vi "Read Settings.vi"() -> (2 "Poly VI Paths":path[](array[path]), 3 "Settings":T1)   [LabVIEW 2020, in "Data Type Scripting.lvlib"]
uses:
  Data Type Scripting.lvlib
  _td_cluster_Settings.ctl
  <vilib>/Utility/config.llb/Read Key (Path).vi
  <vilib>/Utility/config.llb/Write Key (Path).vi
  <vilib>/Utility/config.llb/NI_LVConfig.lvlib
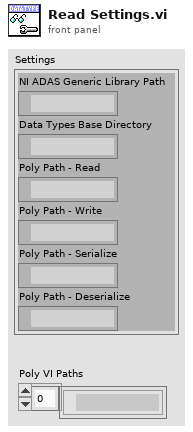
[diagram p1: front panel]
types:
  T1 = typedef "Data Type Scripting.lvlib/_td_cluster_Settings.ctl" = cluster{"NI ADAS Generic Library Path":path, "Data Types Base Directory":path, "Poly Path - Read":path, "Poly Path - Write":path, "Poly Path - Serialize":path, "Poly Path - Deserialize":path}
  T2 = typedef "NI_LVConfig.lvlib/Config Data RefNum.ctl" = refnum<k1>
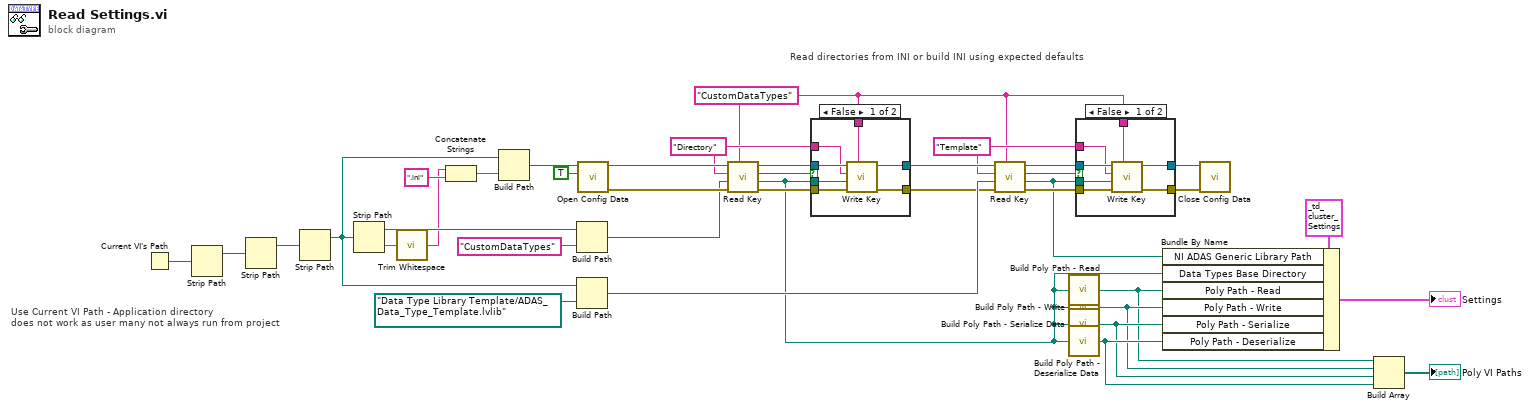
[diagram p0: block diagram]
diagram:
  w7 = "Template" ("key")
  w6 = "CustomDataTypes" ("section")
  w13 = "Directory" ("key")
  # "Read directories from INI or build INI using expected defaults"
  # "Use Current VI Path - Application directory \ndoes not work as user many not always run from project"
  n1 = Current VI's Path() -> (path=w30:path)
  n2 = Strip Path(path=w30) -> (stripped path=w29:path)  [unwired: 1 out]
  n3 = Strip Path(path=w29) -> (stripped path=w28:path)  [unwired: 1 out]
  n4 = Strip Path(path=w28) -> (stripped path=w25:path)  [unwired: 1 out]
  n5 = Strip Path(path=w25) -> (stripped path=w27:path, name=w2:string)
  n6 = call <vilib>:"Trim Whitespace.vi"("string"=w2) -> ("trimmed string"=w1:string)  [unwired: 1 in]
  n7 = Concatenate Strings(w1, ".ini" ("string")) -> (w23:string)
  n8 = Build Path(base path=w25, name or relative path=w23) -> (appended path=w22:path)
  n9 = Build Path(base path=w27, name or relative path="CustomDataTypes") -> (appended path=w19:path)
  n10 = Build Path(base path=w25, name or relative path=path "Data Type Library Template/ADAS_Data_Type_Template.lvlib") -> (appended path=w18:path)
  n11 = call <vilib>:"Open Config Data.vi"("create file if necessary (T)"=TRUE, "configuration file path"=w22) -> ("error out"=w20:errorcluster, "refnum"=w21:T2)  [unwired: 7 in, 1 out]
  n12 = call-poly <vilib>:"Read Key.vi"("section"=w6, "error in (no error)"=w20, "default value"=w19, "key"=w13, "refnum"=w21) -> ("error out"=w16:errorcluster, "value"=w14:path, "found?"=w15:bool, "refnum out"=w17:T2)  [unwired: 3 in]
  n13 = case shown="False" w15 {
    tunnel: w17 -> [w46 w48]
    tunnel: w16 -> [w45 w47]
    tunnel: [w44 w48] -> w12
    tunnel: w6 -> [w43 _]
    tunnel: [w42 w47] -> w11
    tunnel: w14 -> [w41 _]
    tunnel: w13 -> [w40 _]
    frame False {
      n14 = call-poly <vilib>:"Write Key.vi"("section"=w43, "error in (no error)"=w45, "value"=w41, "key"=w40, "refnum"=w46) -> ("error out"=w42:errorcluster, "refnum out"=w44:T2)  [unwired: 4 in, 1 out]
    }
    frame True {
    }
  }
  n15 = call-poly <vilib>:"Read Key.vi"("section"=w6, "error in (no error)"=w11, "default value"=w18, "key"=w7, "refnum"=w12) -> ("error out"=w10:errorcluster, "value"=w8:path, "found?"=w9:bool, "refnum out"=w5:T2)  [unwired: 3 in]
  n16 = call "Build Poly Path - Read.vi"("Directory"=w14) -> ("Path to Read ADAS Data.vi"=w31:path)
  n17 = call "Build Poly Path - Write.vi"("Directory"=w14) -> ("Path to Write ADAS Data.vi"=w32:path)
  n18 = call "Build Poly Path - Serialize Data.vi"("Directory"=w14) -> ("Path to Serialize ADAS Data.vi"=w33:path)
  n19 = call "Build Poly Path - Deserialize Data.vi"("Directory"=w14) -> ("Path to Deserialize ADAS Data.vi"=w34:path)
  n20 = case shown="False" w9 {
    tunnel: w5 -> [w55 w57]
    tunnel: w10 -> [w54 w56]
    tunnel: [w53 w57] -> w4
    tunnel: w6 -> [w52 _]
    tunnel: [w51 w56] -> w3
    tunnel: w8 -> [w50 _]
    tunnel: w7 -> [w49 _]
    frame False {
      n21 = call-poly <vilib>:"Write Key.vi"("section"=w52, "error in (no error)"=w54, "value"=w50, "key"=w49, "refnum"=w55) -> ("error out"=w51:errorcluster, "refnum out"=w53:T2)  [unwired: 4 in, 1 out]
    }
    frame True {
    }
  }
  n22 = Bundle By Name(cluster=T1 {"NI ADAS Generic Library Path"=path "C:/Projects/GitHub/data-record-ad-internal/Data Type Scripting/Data Type Library Template/ADAS_Data_Type_Template.lvlib", "Data Types Base Directory"=path "C:/Projects/GitHub/data-record-ad-internal/Data Types", "Poly Path - Read"=path "C:/Projects/GitHub/data-record-ad-internal/Data Types/Read ADAS Data.vi", "Poly Path - Write"=path "C:/Projects/GitHub/data-record-ad-internal/Data Types/Write ADAS Data.vi", "Poly Path - Serialize"=path "C:/Projects/GitHub/data-record-ad-internal/Data Types/Serialize ADAS Data.vi", "Poly Path - Deserialize"=path "C:/Projects/GitHub/data-record-ad-internal/Data Types/Deserialize ADAS Data.vi"} ("Settings"), "NI ADAS Generic Library Path"=w8, "Data Types Base Directory"=w14, "Poly Path - Read"=w31, "Poly Path - Write"=w32, "Poly Path - Serialize"=w33, "Poly Path - Deserialize"=w34) -> (→"Settings":T1)
  n23 = call <vilib>:"Close Config Data.vi"("error in (no error)"=w3, "refnum"=w4) -> ()  [unwired: 8 in, 2 out]
  n24 = Build Array(w31, w32, w33, w34) -> (→"Poly VI Paths":path[])
